vi "Ping ICPDAS ET7000 modules an UDP.vi"(8 "error in (no error)":errorcluster, 9 "timeout ms (100)":i32=100, 10 "Request":string="ICPDAS7188E,00\r", 11 "IP addr":string="255.255.255.255") -> (0 "error out":errorcluster, 3 "OK":bool)   [LabVIEW 2021, in "TCP.lvclass"]
uses:
  TCP.lvclass
panel:
  out "Name":i32(ring) items=["Empty", "ET-7017-10", "ET-7017-10/PET-7017-10", "ET-7018Z", "ET-7024/PET-7024", "ET-7051", "ET-7051/PET-7051", "PM-3112", "i-7188EX"]
  out "Array":string[](array[string])
  # "Protocol"
  # "Version"
  # "NAME"
  # "ALIAS"
  # "LOCK"
  # "DHCP"
  # "IP"
  # "MASK"
  # "GATEWAY"
  # "MAC"
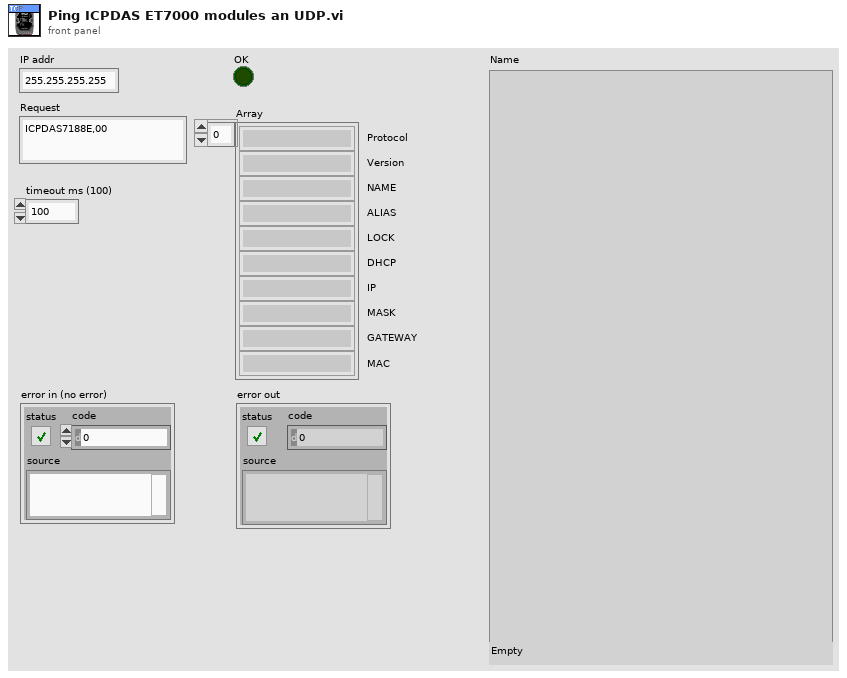
[diagram p1: front panel]
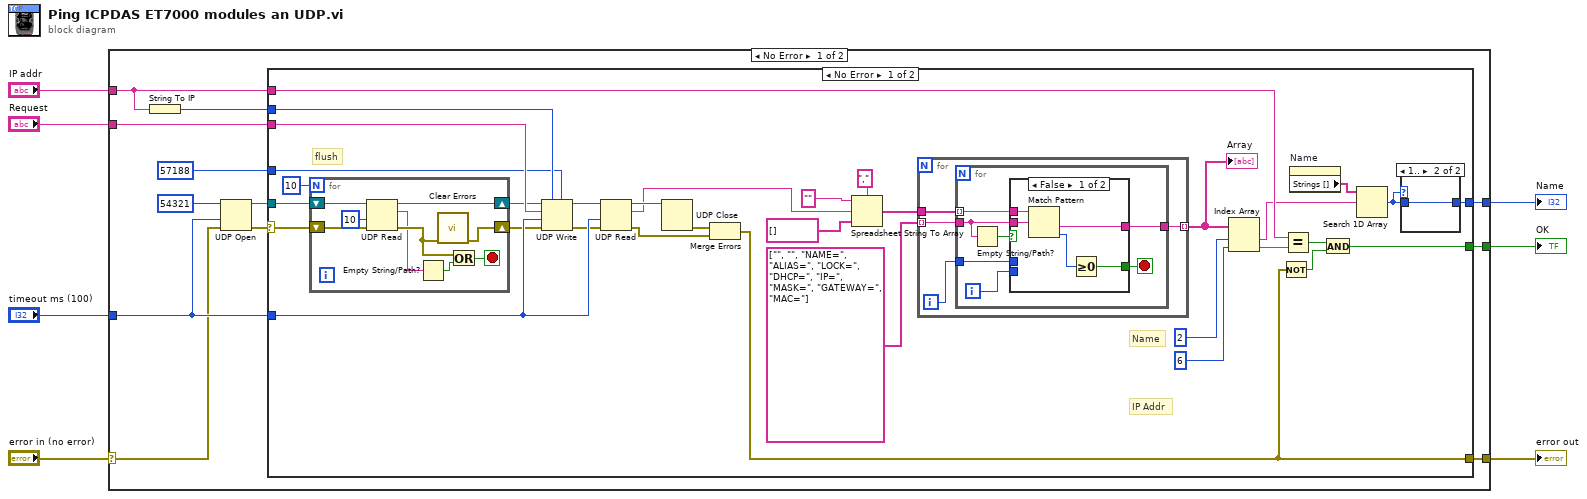
[diagram p0: block diagram]
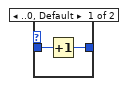
[diagram p2: hidden frame]
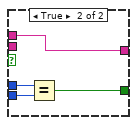
[diagram p3: hidden frame]
diagram:
  n1 = case shown="No Error" "error in (no error)" {
    selector: "error in (no error)" -> [w12 w86]
    tunnel: "Request" -> [w19 _]
    tunnel: "timeout ms (100)" -> [w16 _]
    tunnel: "IP addr" -> [w14 _]
    tunnel: [w13 w86] -> w4
    tunnel: [w11 _] -> w2
    tunnel: [w8 _] -> w1
    frame No Error {
      n2 = String To IP(1:w14) -> (0:w18:u32)
      n3 = UDP Open(8:w12, 9:w16, 11:u16 54321 ("port")) -> (port=w10:refnum<k16>, 0:w9:errorcluster)  [unwired: 2 in, 1 out]
      n4 = case shown="No Error" w9 {
        selector: w9 -> [w33 w85]
        tunnel: w19 -> [w49 _]
        tunnel: w18 -> [w48 _]
        tunnel: u16 57188 ("port") -> [w47 _]
        tunnel: w16 -> [w46 _]
        tunnel: w14 -> [w39 _]
        tunnel: [w37 w85] -> w13
        tunnel: [w26 _] -> w11
        tunnel: w10 -> [w35 _]
        tunnel: [w25 _] -> w8
        frame No Error {
          # "Name"
          # "flush"
          # "IP Addr"
          n5 = for {
            N: 10 -> [_]
            shift-right: [w63] -> w34
            shift-left: w35 -> [w64]
            shift-right: [w60] -> w31
            shift-left: w33 -> [w61]
            stop <- w56 stop-if-true
            n6 = UDP Read(connection ID=w64, timeout ms (25000)=10, 8:w61) -> (data out=w58:string, error out=w59:errorcluster, 3:w63:refnum<k16>)  [unwired: 1 in, 2 out]
            n7 = Empty String/Path?(string/path=w58) -> (empty?=w57:bool)
            n8 = call <vilib>:"Clear Errors.vi"("error in (no error)"=w59) -> ("error out"=w60:errorcluster)  [unwired: 5 in, 1 out]
            n9 = Or(x=w59, y=w57) -> (x .or. y?=w56:bool)
          }
          n10 = UDP Write(address=w48, port or service name=w47, connection ID=w34, data in=w49, 8:w31, 9:w46) -> (error out=w45:errorcluster, 3:w44:refnum<k16>)
          n11 = UDP Read(connection ID=w44, timeout ms (25000)=w46, 8:w45) -> (data out=w23:string, error out=w50:errorcluster, 3:w52:refnum<k16>)  [unwired: 1 in, 2 out]
          n12 = UDP Close(connection ID=w52) -> (error out=w51:errorcluster)  [unwired: 1 in, 1 out]
          n13 = Merge Errors(w51, w50) -> (w37:errorcluster)
          n14 = Spreadsheet String To Array(delimiter (Tab)=",", format string="", spreadsheet string=w23, array type (2D Dbl)=string[] []) -> (array=w22:string[])
          n15 = for {
            tunnel: string[] ["", "", "NAME=", "ALIAS=", "LOCK=", "DHCP=", "IP=", "MASK=", "GATEWAY=", "MAC="] -> [w66] mode=indexing
            tunnel: w22 -> [w68]
            tunnel: [w67] -> w21 mode=indexing
            i -> [w65]
            n16 = for {
              tunnel: w68 -> [w75] mode=indexing
              tunnel: w65 -> [w73]
              tunnel: [w71] -> w67
              tunnel: w66 -> [w70]
              i -> [w69]
              stop <- w72 stop-if-true
              n17 = Empty String/Path?(string/path=w70) -> (empty?=w74:bool)
              n18 = case shown="False" w74 {
                tunnel: w70 -> [w80 _]
                tunnel: w75 -> [w79 w84]
                tunnel: [w78 w84] -> w71
                tunnel: w69 -> [_ w83]
                tunnel: w73 -> [_ w82]
                tunnel: [w77 w81] -> w72
                frame False {
                  n19 = Match Pattern(string=w79, regular expression=w80) -> (after substring=w78:string, offset past match=w76:i32)  [unwired: 1 in, 2 out]
                  n20 = Greater Or Equal To 0?(x=w76) -> (x >= 0?=w77:bool)
                }
                frame True {
                  n21 = Equal?(x=w82, y=w83) -> (x = y?=w81:bool)
                }
              }
            }
          }
          "Array" <- w21
          n22 = Index Array(array=w21, index #1=2 ("index"), index #2=6 ("index")) -> (element #1=w27:string, element #2=w28:string)
          n23 = Not(x=w37) -> (.not. x?=w36:bool)
          n24 = Equal?(x=w39, y=w28) -> (x = y?=w38:bool)
          n25 = property on="Name" class="Ring (strict)"() -> ("Strings []"=w24:string[])  [unwired: 2 in, 2 out]
          n26 = And(x=w38, y=w36) -> (x .and. y?=w26:bool)
          n27 = Search 1D Array(1D array=w24, element=w27) -> (index of element=w20:i32)  [unwired: 1 in]
          n28 = case shown="1.." w20 {
            tunnel: [w54 w55] -> w25
            tunnel: w20 -> [w53 w55]
            frame ..0, Default {
              n29 = Increment(x=w53) -> (x+1=w54:i32)
            }
            frame 1.. {
            }
          }
        }
        frame Error {
        }
      }
    }
    frame Error {
    }
  }
  "error out" <- w4
  "OK" <- w2
  "Name" <- w1
